vi "IsValid2000.vi"   [LabVIEW 2013]
uses:
  <vilib>/Heliosphere Research LLC/Advanced Plotting Toolkit/Advanced Plotting Toolkit.lvlib
types:
  T1 = typedef "Advanced Plotting Toolkit.lvlib/PlotID.ctl" = i32
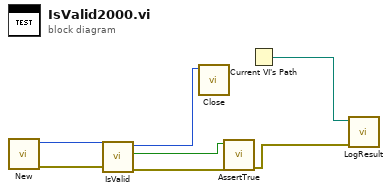
[diagram p0: block diagram]
diagram:
  n1 = call <vilib>:"New.vi"() -> ("error out"=w5:errorcluster, "Plot ID"=w6:T1)  [unwired: 10 in]
  n2 = call <vilib>:"IsValid.vi"("error in (no error)"=w5, "Plot ID"=w6) -> ("error out"=w3:errorcluster, "Valid?"=w1:bool, "Plot ID Out"=w4:T1)  [unwired: 7 in]
  n3 = call <vilib>:"Close.vi"("Plot ID"=w4) -> ()  [unwired: 11 in]
  n4 = call "AssertTrue.vi"("error in (no error)"=w3, "Value"=w1) -> ("error out"=w2:errorcluster)  [unwired: 9 in]
  n5 = Current VI's Path() -> (path=w7:path)
  n6 = call "LogResult.vi"("Test Result"=w2, "VI Path"=w7) -> ()  [unwired: 10 in]
